vi "CRYCalculation TS Tree RowNum.vi"(0 "Tree Task SequenceIn":refnum<vi>, 5 "sOption":string) -> (3 "DispInfo Cluster Out":T1, 4 "Tree Task Sequence Out":refnum<vi>, 6 "SourceRowNum":i32, 8 "SourceCount":i32, 10 "TargetRowNum":i32, 14 "MoveCount":i32, 15 "EditRowNum":i32)   [LabVIEW 2013]
uses:
  CRYProject Editor Global.vi
panel:
  # "Insert new step into Project window."
  # "for Tree"
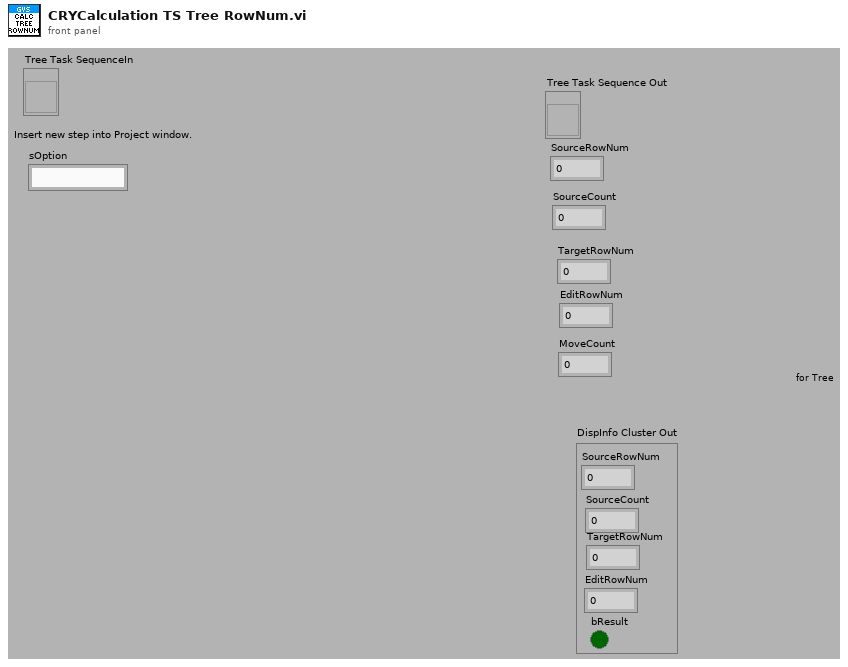
[diagram p1: front panel]
types:
  T1 = cluster{"SourceRowNum":i32, "SourceCount":i32, "TargetRowNum":i32, "bResult":bool, "EditRowNum":i32}
  T2 = typedef "CRYTS.ctl" = cluster{"No.TS":u16, "TS File Path":path, "TS Name":string, "EditStepName":string, "Steps":T3[], "New State":bool, "Change State":bool, "Flattened CurveLib Data":string, "Document Data":string, "EditStepNo":u16, "Operator Start File":string, "Sequence Type":string, "Sequence Language":string}
  T3 = typedef "CRYStep.ctl" = cluster{"No.VI":i32, "Category":string, "StepName":string, "Seq setup flattened":string, "Comment":string, "Steps config.":bool[], "Jump config":i32[], "Start":dbl, "Increment":dbl, "Name":string, "Unit":string, "Y data":u16, "Y prefix":string, "Y dB ref":dbl, "Y unit":string, "Repeat State Array":cluster{"Start":dbl, "Increment":dbl, "Count":i32, "Num":i32}[]}
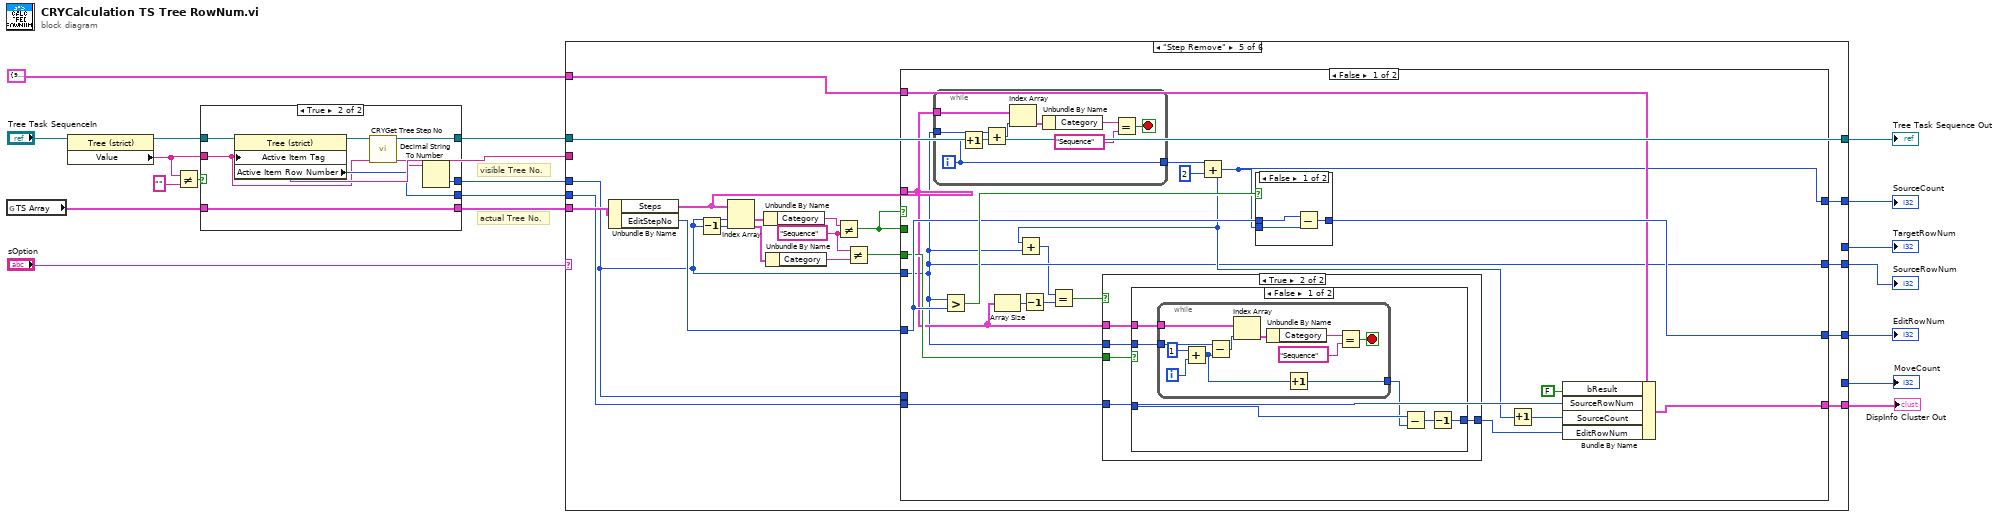
[diagram p0: block diagram]
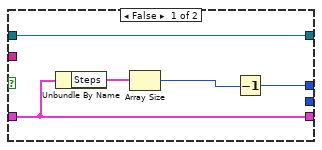
[diagram p2: hidden frame]
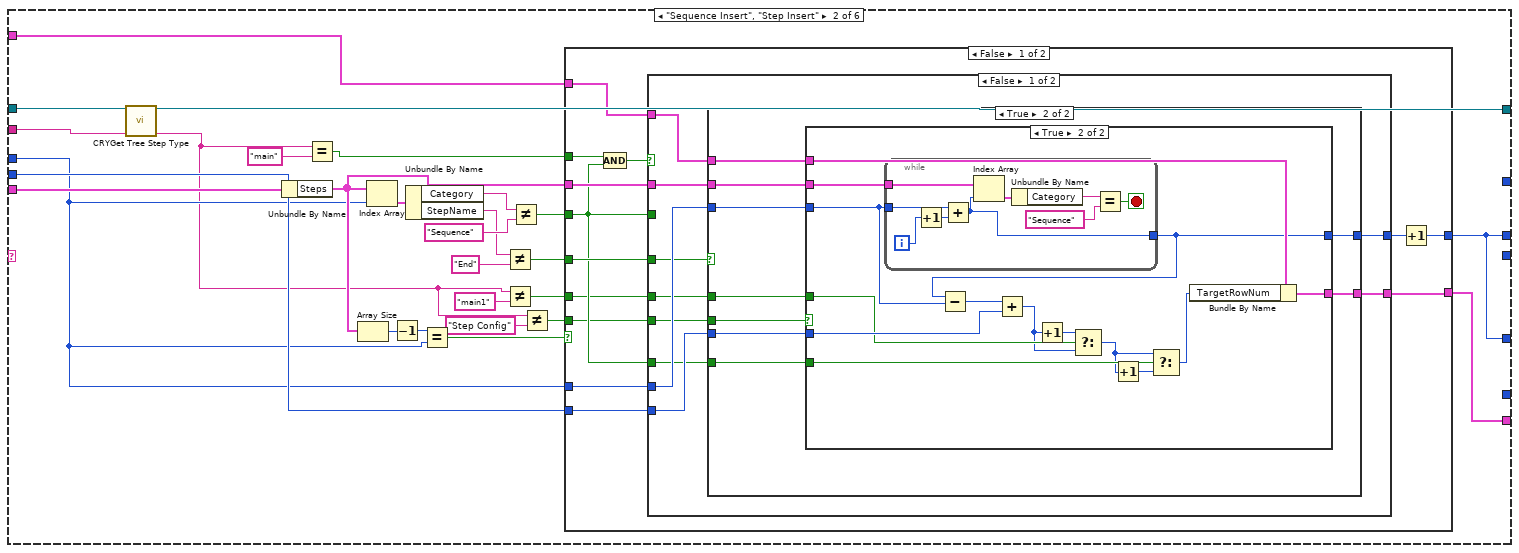
[diagram p4: hidden frame]
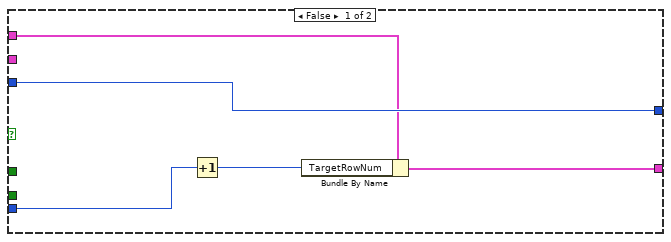
[diagram p5: hidden frame]
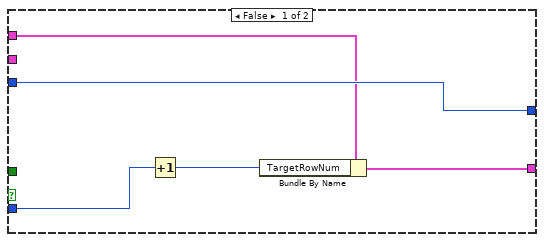
[diagram p6: hidden frame]
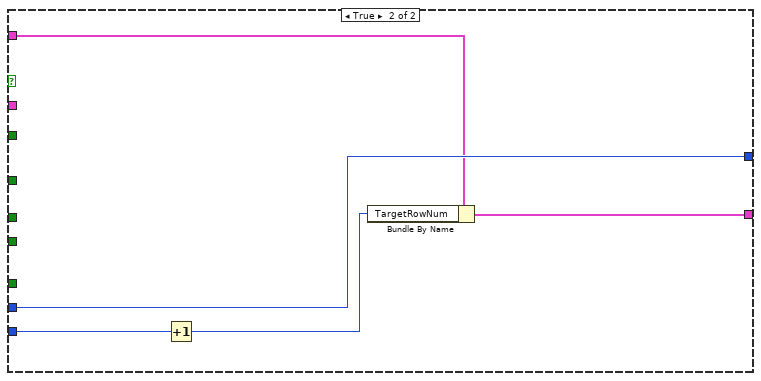
[diagram p7: hidden frame]
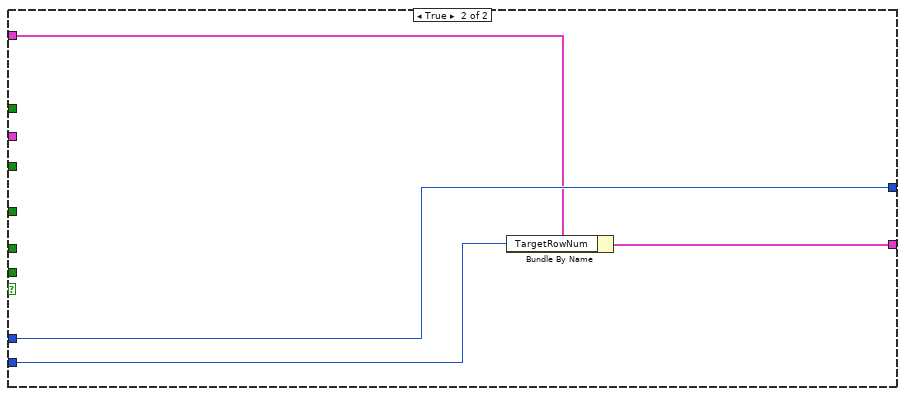
[diagram p8: hidden frame]
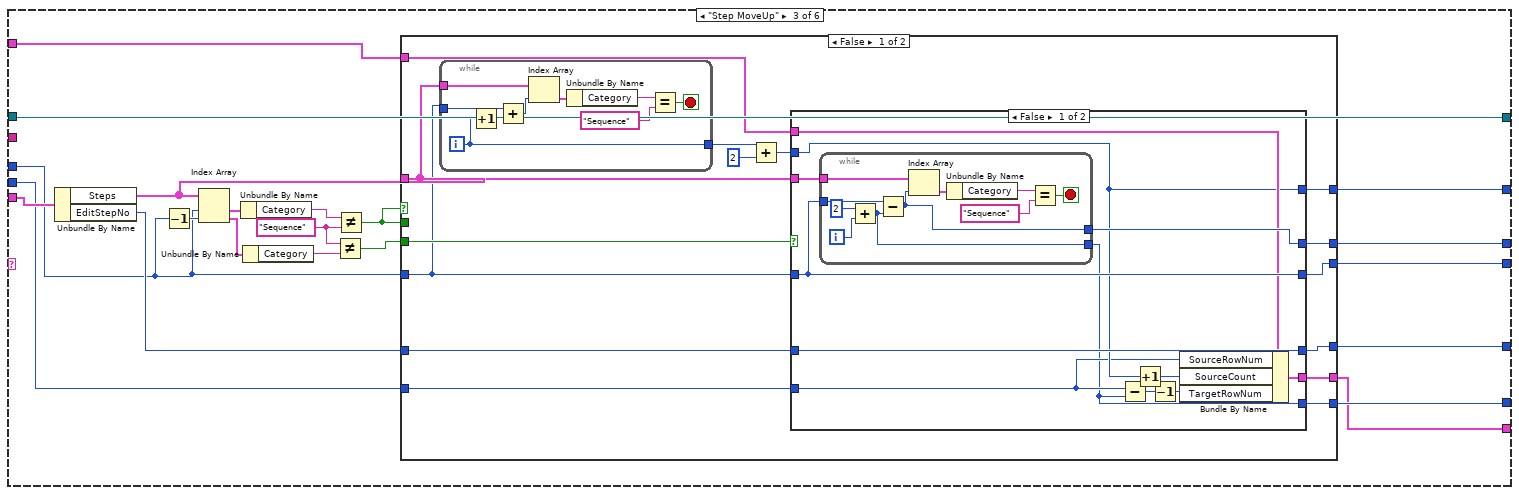
[diagram p9: hidden frame]
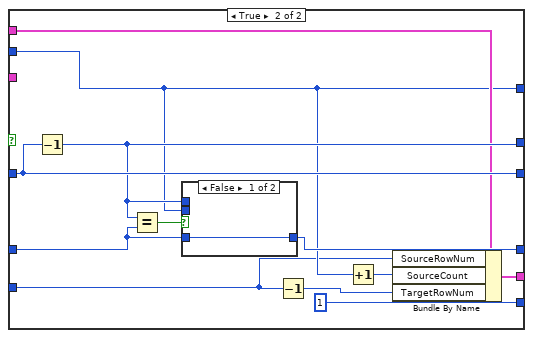
[diagram p10: hidden frame]
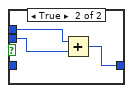
[diagram p11: hidden frame]
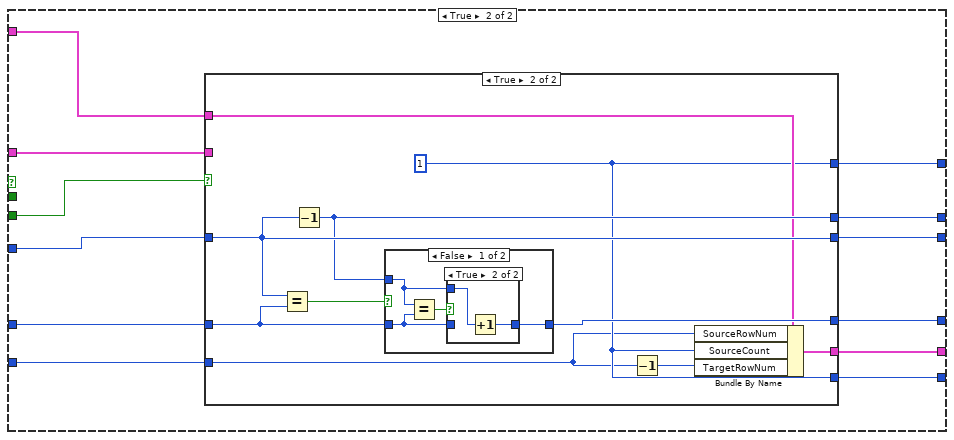
[diagram p12: hidden frame]
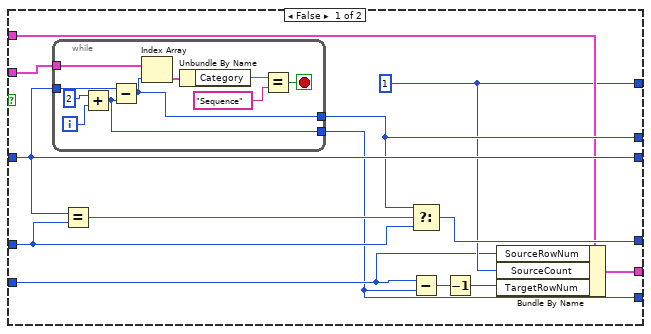
[diagram p13: hidden frame]
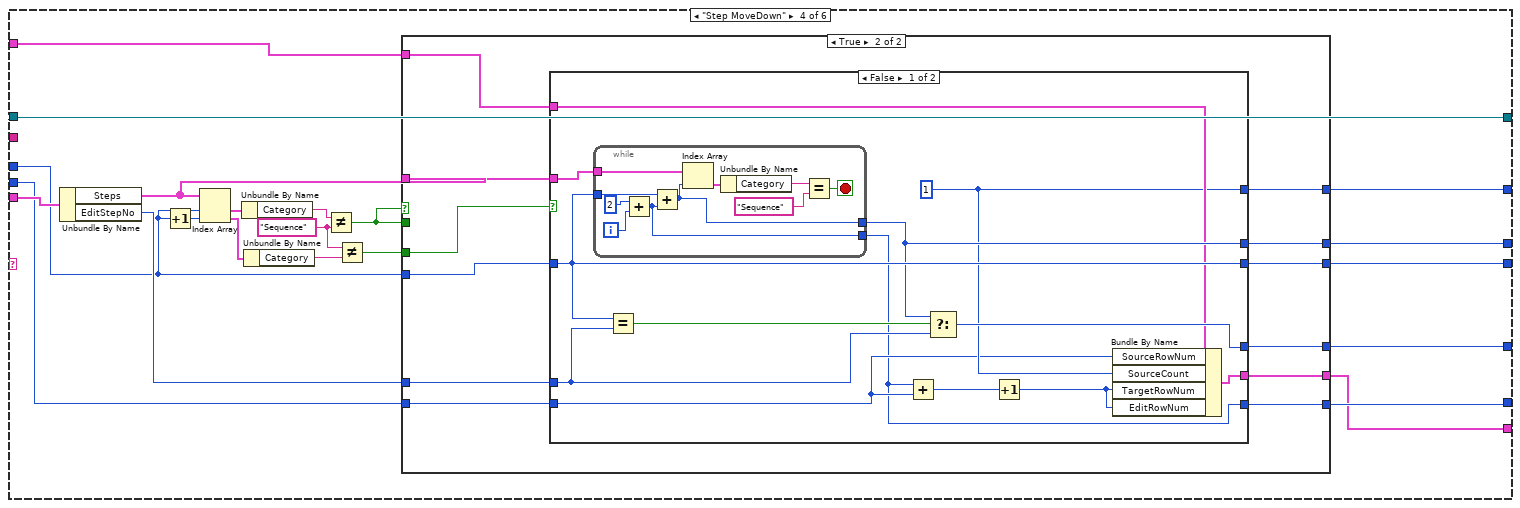
[diagram p16: hidden frame]
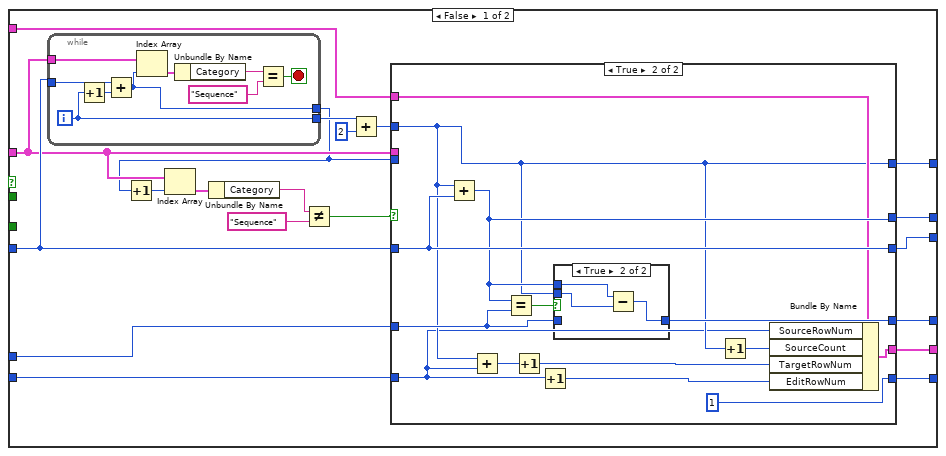
[diagram p17: hidden frame]
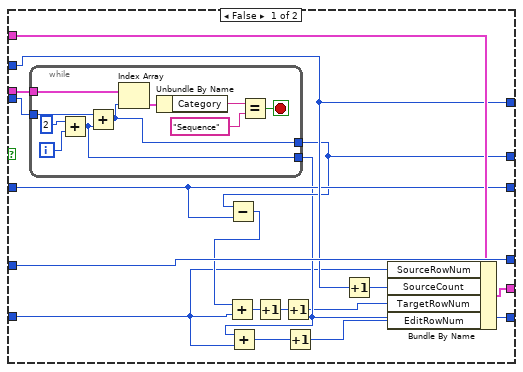
[diagram p18: hidden frame]
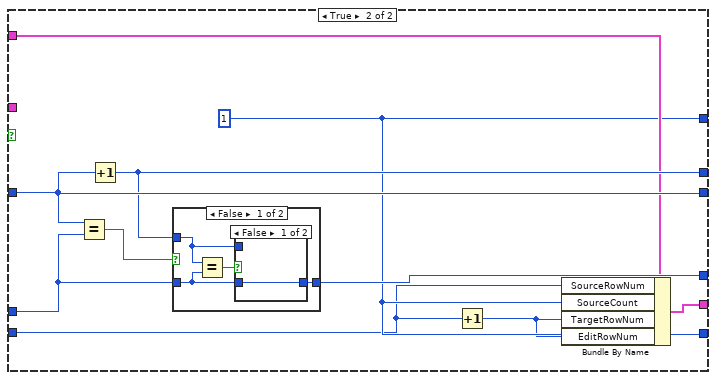
[diagram p20: hidden frame]
diagram:
  # "actual Tree No."
  # "visible Tree No."
  n1 = global read "CRYProject Editor Global.vi" "TS Array"() -> (w2:T2)
  n2 = property class="Tree (strict)"(reference="Tree Task SequenceIn") -> (reference out=w7:refnum<vi>, "Value"=w5:string)  [unwired: 1 in, 1 out]
  n3 = Not Equal?(x=w5, y="") -> (x != y?=w3:bool)
  n4 = case shown="True" w3 {
    tunnel: [w22 w32] -> w9
    tunnel: [_ w31] -> w8
    tunnel: w7 -> [w20 w29]
    tunnel: [w20 w27] -> w6
    tunnel: w5 -> [_ w26]
    tunnel: w2 -> [w21 w25]
    tunnel: [w21 w25] -> w1
    frame False {
      n5 = Unbundle By Name(w21) -> ("Steps"=w24:T3[])
      n6 = Array Size(array=w24) -> (size(s)=w23:i32)
      n7 = Decrement(x=w23) -> (x-1=w22:i32)
    }
    frame True {
      n8 = property class="Tree (strict)"(reference=w29, "Active Item Tag"=w26) -> (reference out=w28:refnum<vi>, "Active Item Row Number"=w31:i32)  [unwired: 1 in, 1 out]
      n9 = call "CRYGet Tree Step No.vi"("SequenceTree"=w28, "Active Item Tag"=w26) -> ("reference out"=w27:refnum<vi>, "Active Cell String4"=w30:string)  [unwired: 12 in]
      n10 = Decimal String To Number(string=w30) -> (number=w32:i32)  [unwired: 2 in, 1 out]
    }
  }
  n11 = case shown="\"Step Remove\"" "sOption" {
    tunnel: w6 -> [w33 w37 w135 w271 w420 w699]
    tunnel: [w33 w36 w135 w271 w420 w699] -> w19
    tunnel: [_ w49 w152 w288 _ _] -> w17
    tunnel: [_ _ w145 w281 w428 _] -> w16
    tunnel: [_ _ w144 w280 w427 _] -> w15
    tunnel: [_ w49 w143 w278 w425 _] -> w14
    tunnel: [_ _ w141 w277 _ _] -> w13
    tunnel: [_ w47 w139 w275 w424 w697] -> w12
    tunnel: T1 {"SourceRowNum"=9, "SourceCount"=19, "TargetRowNum"=42, "bResult"=FALSE, "EditRowNum"=42} ("DispInfo Cluster Out") -> [_ w48 w140 w276 w423 w698]
    tunnel: w1 -> [_ w42 w138 w274 w422 _]
    tunnel: w9 -> [_ w40 w136 w272 w419 w696]
    tunnel: w8 -> [_ w41 w137 w273 w421 _]
    tunnel: w5 -> [_ w35 _ _ _ _]
    frame Default {
    }
    frame "Sequence Insert", "Step Insert" {
      n12 = call "CRYGet Tree Step Type.vi"("SequenceTree"=w37, "Active Item Tag"=w35) -> ("reference out"=w36:refnum<vi>, "Active Cell String3"=w34:string)  [unwired: 12 in]
      n13 = Unbundle By Name(w42) -> ("Steps"=w55:T3[])
      n14 = Equal?(x=w34, y="main" ("decimal integer string")) -> (x = y?=w57:bool)
      n15 = Array Size(array=w55) -> (size(s)=w54:i32)
      n16 = Index Array(array=w55, index=w40) -> (element=w60:T3)
      n17 = Decrement(x=w54) -> (x-1=w53:i32)
      n18 = Unbundle By Name(w60) -> ("Category"=w59:string, "StepName"=w46:string)
      n19 = Equal?(x=w53, y=w40) -> (x = y?=w52:bool)
      n20 = Not Equal?(x=w46, y="End") -> (x != y?=w50:bool)
      n21 = Not Equal?(x=w34, y="main1" ("decimal integer string")) -> (x != y?=w45:bool)
      n22 = Not Equal?(x=w59, y="Sequence") -> (x != y?=w56:bool)
      n23 = Not Equal?(x=w34, y="Step Config" ("SequenceName")) -> (x != y?=w38:bool)
      n24 = case shown="False" w52 {
        tunnel: w57 -> [w73 _]
        tunnel: w56 -> [w63 _]
        tunnel: [w70 w134] -> w49
        tunnel: w55 -> [w69 _]
        tunnel: w40 -> [w68 w134]
        tunnel: w50 -> [w67 _]
        tunnel: w48 -> [w66 w133]
        tunnel: w41 -> [w65 w132]
        tunnel: [w64 w131] -> w47
        tunnel: w45 -> [w62 _]
        tunnel: w38 -> [w61 _]
        frame False {
          n25 = Compound Arithmetic op=AND(w73, w63) -> (w72:bool)
          n26 = case shown="False" w72 {
            tunnel: w68 -> [w83 w130]
            tunnel: w63 -> [_ _]
            tunnel: w69 -> [w82 _]
            tunnel: [w81 w130] -> w71
            tunnel: w67 -> [w80 _]
            tunnel: w66 -> [w79 w129]
            tunnel: w65 -> [w78 w128]
            tunnel: [w77 w127] -> w64
            tunnel: w63 -> [w76 _]
            tunnel: w62 -> [w75 _]
            tunnel: w61 -> [w74 _]
            frame False {
              n27 = case shown="True" w80 {
                tunnel: w83 -> [w88 w93]
                tunnel: w82 -> [_ w97]
                tunnel: [w88 w94] -> w81
                tunnel: w79 -> [w87 w96]
                tunnel: w78 -> [w86 w92]
                tunnel: [w85 w95] -> w77
                tunnel: w76 -> [_ w91]
                tunnel: w75 -> [_ w90]
                tunnel: w74 -> [_ w89]
                frame False {
                  n28 = Increment(x=w86) -> (x+1=w84:i32)
                  n29 = Bundle By Name(cluster=w87, "TargetRowNum"=w84) -> (w85:T1)
                }
                frame True {
                  n30 = case shown="True" w89 {
                    tunnel: w97 -> [_ w116]
                    tunnel: w96 -> [w100 w115]
                    tunnel: [w98 w114] -> w95
                    tunnel: [w101 w113] -> w94
                    tunnel: w93 -> [w101 w112]
                    tunnel: w92 -> [w99 w110]
                    tunnel: w91 -> [_ w109]
                    tunnel: w90 -> [_ w106]
                    frame False {
                      n31 = Increment(x=w99) -> (x+1=w102:i32)
                      n32 = Bundle By Name(cluster=w100, "TargetRowNum"=w102) -> (w98:T1)
                    }
                    frame True {
                      n33 = while {
                        tunnel: w116 -> [w125]
                        tunnel: w112 -> [w124]
                        tunnel: [w117] -> w113
                        i -> [w123]
                        stop <- w118 stop-if-true
                        n34 = Increment(x=w123) -> (x+1=w122:i32)
                        n35 = Add(x=w124, y=w122) -> (x+y=w117:i32)
                        n36 = Index Array(array=w125, index=w117) -> (element=w121:T3)
                        n37 = Unbundle By Name(w121) -> ("Category"=w120:string)
                        n38 = Equal?(x=w120, y="Sequence") -> (x = y?=w118:bool)
                      }
                      n39 = Subtract(x=w113, y=w112) -> (x-y=w111:i32)
                      n40 = Add(x=w111, y=w110) -> (x+y=w105:i32)
                      n41 = Increment(x=w105) -> (x+1=w104:i32)
                      n42 = Select(t=w104, s=w106, f=w105) -> (s? t:f=w103:i32)
                      n43 = Increment(x=w103) -> (x+1=w108:i32)
                      n44 = Select(t=w103, s=w109, f=w108) -> (s? t:f=w107:i32)
                      n45 = Bundle By Name(cluster=w115, "TargetRowNum"=w107) -> (w114:T1)
                    }
                  }
                }
              }
            }
            frame True {
              n46 = Increment(x=w128) -> (x+1=w126:i32)
              n47 = Bundle By Name(cluster=w129, "TargetRowNum"=w126) -> (w127:T1)
            }
          }
          n48 = Increment(x=w71) -> (x+1=w70:i32)
        }
        frame True {
          n49 = Bundle By Name(cluster=w133, "TargetRowNum"=w132) -> (w131:T1)
        }
      }
    }
    frame "Step MoveUp" {
      w147 = "Sequence" ("y")
      n50 = Unbundle By Name(w138) -> ("Steps"=w153:T3[], "EditStepNo"=w142:u16)
      n51 = Decrement(x=w136) -> (x-1=w150:i32)
      n52 = Index Array(array=w153, index #1=w136, index #2=w150) -> (element #1=w155:T3, element #2=w149:T3)
      n53 = Unbundle By Name(w155) -> ("Category"=w154:string)
      n54 = Unbundle By Name(w149) -> ("Category"=w148:string)
      n55 = Not Equal?(x=w147, y=w148) -> (x != y?=w146:bool)
      n56 = Not Equal?(x=w154, y=w147) -> (x != y?=w151:bool)
      n57 = case shown="False" w151 {
        tunnel: w136 -> [w165 w228]
        tunnel: w151 -> [_ _]
        tunnel: w153 -> [w166 w226]
        tunnel: [w170 w227] -> w152
        tunnel: w146 -> [w169 w229]
        tunnel: [w168 w225] -> w145
        tunnel: [w167 w224] -> w144
        tunnel: [w160 w223] -> w143
        tunnel: w142 -> [w161 w222]
        tunnel: [w159 w221] -> w141
        tunnel: w140 -> [w158 w220]
        tunnel: w137 -> [w157 w218]
        tunnel: [w156 w219] -> w139
        frame False {
          n58 = while {
            tunnel: w166 -> [w179]
            tunnel: w165 -> [w178]
            tunnel: [w171] -> w163
            i -> [w171]
            stop <- w173 stop-if-true
            n59 = Increment(x=w171) -> (x+1=w177:i32)
            n60 = Add(x=w178, y=w177) -> (x+y=w172:i32)
            n61 = Index Array(array=w179, index=w172) -> (element=w176:T3)
            n62 = Unbundle By Name(w176) -> ("Category"=w175:string)
            n63 = Equal?(x=w175, y="Sequence") -> (x = y?=w173:bool)
          }
          n64 = Add(x=w163, y=2) -> (x+y=w162:i32)
          n65 = case shown="False" w169 {
            tunnel: w166 -> [w191 _]
            tunnel: [w190 w211] -> w170
            tunnel: w165 -> [w189 w213]
            tunnel: [w189 w213] -> w168
            tunnel: [w186 w205] -> w167
            tunnel: w162 -> [w186 w205]
            tunnel: w161 -> [w188 w210]
            tunnel: [w188 w209] -> w160
            tunnel: [w183 1] -> w159
            tunnel: w158 -> [w187 w207]
            tunnel: w157 -> [w184 w203]
            tunnel: [w180 w206] -> w156
            frame False {
              n66 = while {
                tunnel: w191 -> [w201]
                tunnel: w189 -> [w200]
                tunnel: [w195] -> w190
                tunnel: [w192] -> w183
                i -> [w194]
                stop <- w196 stop-if-true
                n67 = Add(x=2, y=w194) -> (x+y=w192:i32)
                n68 = Subtract(x=w200, y=w192) -> (x-y=w195:i32)
                n69 = Index Array(array=w201, index=w195) -> (element=w199:T3)
                n70 = Unbundle By Name(w199) -> ("Category"=w198:string)
                n71 = Equal?(x=w198, y="Sequence") -> (x = y?=w196:bool)
              }
              n72 = Subtract(x=w184, y=w183) -> (x-y=w182:i32)
              n73 = Increment(x=w186) -> (x+1=w185:i32)
              n74 = Decrement(x=w182) -> (x-1=w181:i32)
              n75 = Bundle By Name(cluster=w187, "SourceRowNum"=w184, "SourceCount"=w185, "TargetRowNum"=w181) -> (w180:T1)
            }
            frame True {
              n76 = Decrement(x=w213) -> (x-1=w211:i32)
              n77 = Equal?(x=w211, y=w210) -> (x = y?=w212:bool)
              n78 = case shown="False" w212 {
                tunnel: w211 -> [_ w217]
                tunnel: [w214 w215] -> w209
                tunnel: w210 -> [w214 _]
                tunnel: w205 -> [_ w216]
                frame False {
                }
                frame True {
                  n79 = Add(x=w217, y=w216) -> (x+y=w215:i32)
                }
              }
              n80 = Decrement(x=w203) -> (x-1=w202:i32)
              n81 = Increment(x=w205) -> (x+1=w204:i32)
              n82 = Bundle By Name(cluster=w207, "SourceRowNum"=w203, "SourceCount"=w204, "TargetRowNum"=w202) -> (w206:T1)
            }
          }
        }
        frame True {
          n83 = case shown="True" w229 {
            tunnel: [w239 w260] -> w227
            tunnel: w228 -> [w241 w262]
            tunnel: w226 -> [w242 _]
            tunnel: [w241 w262] -> w225
            tunnel: [w234 w255] -> w224
            tunnel: [w237 w259] -> w223
            tunnel: w222 -> [w238 w258]
            tunnel: [w232 w255] -> w221
            tunnel: w220 -> [w236 w257]
            tunnel: [w235 w256] -> w219
            tunnel: w218 -> [w233 w254]
            frame False {
              w234 = 1 ("x-1")
              n84 = while {
                tunnel: w242 -> [w252]
                tunnel: w241 -> [w251]
                tunnel: [w246] -> w239
                tunnel: [w243] -> w232
                i -> [w245]
                stop <- w247 stop-if-true
                n85 = Add(x=2, y=w245) -> (x+y=w243:i32)
                n86 = Subtract(x=w251, y=w243) -> (x-y=w246:i32)
                n87 = Index Array(array=w252, index=w246) -> (element=w250:T3)
                n88 = Unbundle By Name(w250) -> ("Category"=w249:string)
                n89 = Equal?(x=w249, y="Sequence") -> (x = y?=w247:bool)
              }
              n90 = Equal?(x=w241, y=w238) -> (x = y?=w240:bool)
              n91 = Select(t=w239, s=w240, f=w238) -> (s? t:f=w237:i32)
              n92 = Subtract(x=w233, y=w232) -> (x-y=w231:i32)
              n93 = Decrement(x=w231) -> (x-1=w230:i32)
              n94 = Bundle By Name(cluster=w236, "SourceRowNum"=w233, "SourceCount"=w234, "TargetRowNum"=w230) -> (w235:T1)
            }
            frame True {
              w255 = 1 ("x-1")
              n95 = Equal?(x=w262, y=w258) -> (x = y?=w261:bool)
              n96 = Decrement(x=w262) -> (x-1=w260:i32)
              n97 = case shown="False" w261 {
                tunnel: [w264 w270] -> w259
                tunnel: w260 -> [w265 w270]
                tunnel: w258 -> [w263 _]
                frame False {
                  n98 = Equal?(x=w265, y=w263) -> (x = y?=w266:bool)
                  n99 = case shown="True" w266 {
                    tunnel: w265 -> [_ w269]
                    tunnel: [w267 w268] -> w264
                    tunnel: w263 -> [w267 _]
                    frame False {
                    }
                    frame True {
                      n100 = Increment(x=w269) -> (x+1=w268:i32)
                    }
                  }
                }
                frame True {
                }
              }
              n101 = Decrement(x=w254) -> (x-1=w253:i32)
              n102 = Bundle By Name(cluster=w257, "SourceRowNum"=w254, "SourceCount"=w255, "TargetRowNum"=w253) -> (w256:T1)
            }
          }
        }
      }
    }
    frame "Step MoveDown" {
      w283 = "Sequence" ("y")
      n103 = Unbundle By Name(w274) -> ("Steps"=w289:T3[], "EditStepNo"=w279:u16)
      n104 = Increment(x=w272) -> (x+1=w286:i32)
      n105 = Index Array(array=w289, index #1=w272, index #2=w286) -> (element #1=w291:T3, element #2=w285:T3)
      n106 = Unbundle By Name(w291) -> ("Category"=w290:string)
      n107 = Unbundle By Name(w285) -> ("Category"=w284:string)
      n108 = Not Equal?(x=w290, y=w283) -> (x != y?=w287:bool)
      n109 = Not Equal?(x=w283, y=w284) -> (x != y?=w282:bool)
      n110 = case shown="True" w287 {
        tunnel: w272 -> [w308 w376]
        tunnel: w287 -> [_ _]
        tunnel: w289 -> [w301 w374]
        tunnel: [w311 w375] -> w288
        tunnel: w282 -> [_ w377]
        tunnel: [w310 w373] -> w281
        tunnel: [w309 w372] -> w280
        tunnel: w279 -> [w305 w371]
        tunnel: [w304 w370] -> w278
        tunnel: [w303 w369] -> w277
        tunnel: w276 -> [w294 w368]
        tunnel: w273 -> [w293 w366]
        tunnel: [w292 w367] -> w275
        frame False {
          n111 = while {
            tunnel: w301 -> [w320]
            tunnel: w308 -> [w319]
            tunnel: [w313] -> w300
            tunnel: [w312] -> w295
            i -> [w313]
            stop <- w314 stop-if-true
            n112 = Increment(x=w313) -> (x+1=w318:i32)
            n113 = Add(x=w319, y=w318) -> (x+y=w312:i32)
            n114 = Index Array(array=w320, index=w312) -> (element=w317:T3)
            n115 = Unbundle By Name(w317) -> ("Category"=w316:string)
            n116 = Equal?(x=w316, y="Sequence") -> (x = y?=w314:bool)
          }
          n117 = Increment(x=w295) -> (x+1=w299:i32)
          n118 = Index Array(array=w301, index=w299) -> (element=w302:T3)
          n119 = Unbundle By Name(w302) -> ("Category"=w298:string)
          n120 = Not Equal?(x=w298, y="Sequence") -> (x != y?=w296:bool)
          n121 = Add(x=w300, y=2) -> (x+y=w306:i32)
          n122 = case shown="True" w296 {
            tunnel: w301 -> [w337 _]
            tunnel: [w327 w356] -> w311
            tunnel: w308 -> [w329 w358]
            tunnel: [w329 w358] -> w310
            tunnel: [w332 w352] -> w309
            tunnel: w306 -> [w332 w352]
            tunnel: [w336 w360] -> w304
            tunnel: w305 -> [w336 w361]
            tunnel: [w326 1] -> w303
            tunnel: w295 -> [w335 _]
            tunnel: w294 -> [w334 w355]
            tunnel: w293 -> [w325 w349]
            tunnel: [w333 w353] -> w292
            frame False {
              n123 = while {
                tunnel: w337 -> [w347]
                tunnel: w335 -> [w346]
                tunnel: [w341] -> w327
                tunnel: [w338] -> w326
                i -> [w340]
                stop <- w342 stop-if-true
                n124 = Add(x=2, y=w340) -> (x+y=w338:i32)
                n125 = Add(x=w346, y=w338) -> (x+y=w341:i32)
                n126 = Index Array(array=w347, index=w341) -> (element=w345:T3)
                n127 = Unbundle By Name(w345) -> ("Category"=w344:string)
                n128 = Equal?(x=w344, y="Sequence") -> (x = y?=w342:bool)
              }
              n129 = Subtract(x=w327, y=w329) -> (x-y=w328:i32)
              n130 = Add(x=w328, y=w325) -> (x+y=w330:i32)
              n131 = Add(x=w326, y=w325) -> (x+y=w322:i32)
              n132 = Increment(x=w330) -> (x+1=w324:i32)
              n133 = Increment(x=w324) -> (x+1=w323:i32)
              n134 = Increment(x=w322) -> (x+1=w321:i32)
              n135 = Increment(x=w332) -> (x+1=w331:i32)
              n136 = Bundle By Name(cluster=w334, "SourceRowNum"=w325, "SourceCount"=w331, "TargetRowNum"=w323, "EditRowNum"=w321) -> (w333:T1)
            }
            frame True {
              n137 = Add(x=w352, y=w358) -> (x+y=w356:i32)
              n138 = Add(x=w352, y=w349) -> (x+y=w351:i32)
              n139 = Equal?(x=w356, y=w361) -> (x = y?=w359:bool)
              n140 = Increment(x=w351) -> (x+1=w350:i32)
              n141 = Increment(x=w349) -> (x+1=w348:i32)
              n142 = case shown="True" w359 {
                tunnel: w356 -> [_ w365]
                tunnel: [w362 w363] -> w360
                tunnel: w361 -> [w362 _]
                tunnel: w352 -> [_ w364]
                frame False {
                }
                frame True {
                  n143 = Subtract(x=w365, y=w364) -> (x-y=w363:i32)
                }
              }
              n144 = Increment(x=w352) -> (x+1=w354:i32)
              n145 = Bundle By Name(cluster=w355, "SourceRowNum"=w349, "SourceCount"=w354, "TargetRowNum"=w350, "EditRowNum"=w348) -> (w353:T1)
            }
          }
        }
        frame True {
          n146 = case shown="False" w377 {
            tunnel: [w385 w406] -> w375
            tunnel: w376 -> [w389 w410]
            tunnel: w374 -> [w390 _]
            tunnel: [w389 w410] -> w373
            tunnel: [w382 w403] -> w372
            tunnel: w371 -> [w387 w408]
            tunnel: [w386 w407] -> w370
            tunnel: [w380 w403] -> w369
            tunnel: w368 -> [w384 w405]
            tunnel: [w383 w404] -> w367
            tunnel: w366 -> [w381 w402]
            frame False {
              w382 = 1 ("x-1")
              n147 = while {
                tunnel: w390 -> [w400]
                tunnel: w389 -> [w399]
                tunnel: [w394] -> w385
                tunnel: [w391] -> w380
                i -> [w393]
                stop <- w395 stop-if-true
                n148 = Add(x=2, y=w393) -> (x+y=w391:i32)
                n149 = Add(x=w399, y=w391) -> (x+y=w394:i32)
                n150 = Index Array(array=w400, index=w394) -> (element=w398:T3)
                n151 = Unbundle By Name(w398) -> ("Category"=w397:string)
                n152 = Equal?(x=w397, y="Sequence") -> (x = y?=w395:bool)
              }
              n153 = Equal?(x=w389, y=w387) -> (x = y?=w388:bool)
              n154 = Add(x=w380, y=w381) -> (x+y=w379:i32)
              n155 = Select(t=w385, s=w388, f=w387) -> (s? t:f=w386:i32)
              n156 = Increment(x=w379) -> (x+1=w378:i32)
              n157 = Bundle By Name(cluster=w384, "SourceRowNum"=w381, "SourceCount"=w382, "TargetRowNum"=w378, "EditRowNum"=w378) -> (w383:T1)
            }
            frame True {
              w403 = 1 ("x-1")
              n158 = Equal?(x=w410, y=w408) -> (x = y?=w409:bool)
              n159 = Increment(x=w410) -> (x+1=w406:i32)
              n160 = case shown="False" w409 {
                tunnel: [w412 w418] -> w407
                tunnel: w406 -> [w413 w418]
                tunnel: w408 -> [w411 _]
                frame False {
                  n161 = Equal?(x=w413, y=w411) -> (x = y?=w414:bool)
                  n162 = case shown="False" w414 {
                    tunnel: w413 -> [_ w417]
                    tunnel: [w415 w416] -> w412
                    tunnel: w411 -> [w415 _]
                    frame False {
                    }
                    frame True {
                      n163 = Decrement(x=w417) -> (x-1=w416:i32)
                    }
                  }
                }
                frame True {
                }
              }
              n164 = Increment(x=w402) -> (x+1=w401:i32)
              n165 = Bundle By Name(cluster=w405, "SourceRowNum"=w402, "SourceCount"=w403, "TargetRowNum"=w401, "EditRowNum"=w401) -> (w404:T1)
            }
          }
        }
      }
    }
    frame "Step Remove" {
      w430 = "Sequence" ("y")
      n166 = Unbundle By Name(w422) -> ("Steps"=w435:T3[], "EditStepNo"=w426:u16)
      n167 = Decrement(x=w419) -> (x-1=w433:i32)
      n168 = Index Array(array=w435, index #1=w419, index #2=w433) -> (element #1=w437:T3, element #2=w432:T3)
      n169 = Unbundle By Name(w437) -> ("Category"=w436:string)
      n170 = Unbundle By Name(w432) -> ("Category"=w431:string)
      n171 = Not Equal?(x=w436, y=w430) -> (x != y?=w434:bool)
      n172 = Not Equal?(x=w430, y=w431) -> (x != y?=w429:bool)
      n173 = case shown="False" w434 {
        tunnel: w419 -> [w441 w500]
        tunnel: w434 -> [_ _]
        tunnel: w435 -> [w444 w499]
        tunnel: w429 -> [w446 w498]
        tunnel: [w441 w500] -> w428
        tunnel: [w442 w501] -> w427
        tunnel: w426 -> [w453 w506]
        tunnel: [w452 w508] -> w425
        tunnel: [w449 w504] -> w424
        tunnel: w423 -> [w451 w503]
        tunnel: w421 -> [w447 w497]
        tunnel: w419 -> [_ w495]
        frame False {
          n174 = while {
            tunnel: w444 -> [w494]
            tunnel: w441 -> [w493]
            tunnel: [w486] -> w455
            i -> [w486]
            stop <- w488 stop-if-true
            n175 = Increment(x=w486) -> (x+1=w492:i32)
            n176 = Add(x=w493, y=w492) -> (x+y=w487:i32)
            n177 = Index Array(array=w494, index=w487) -> (element=w491:T3)
            n178 = Unbundle By Name(w491) -> ("Category"=w490:string)
            n179 = Equal?(x=w490, y="Sequence") -> (x = y?=w488:bool)
          }
          n180 = Greater?(x=w441, y=w453) -> (0:w454:bool)
          n181 = Array Size(array=w444) -> (size(s)=w443:i32)
          n182 = Decrement(x=w443) -> (x-1=w440:i32)
          n183 = Add(x=w455, y=2) -> (x+y=w442:i32)
          n184 = Add(x=w442, y=w441) -> (x+y=w439:i32)
          n185 = Equal?(x=w439, y=w440) -> (x = y?=w438:bool)
          n186 = case shown="True" w438 {
            tunnel: w447 -> [w457 w462]
            tunnel: w446 -> [_ w461]
            tunnel: [w457 w460] -> w445
            tunnel: w444 -> [_ w459]
            tunnel: w441 -> [_ w458]
            frame False {
            }
            frame True {
              n187 = case shown="False" w461 {
                tunnel: w459 -> [w468 _]
                tunnel: w458 -> [w467 _]
                tunnel: w462 -> [w466 w481]
                tunnel: [w463 w480] -> w460
                frame False {
                  n188 = while {
                    tunnel: w468 -> [w479]
                    tunnel: w467 -> [w478]
                    tunnel: [w469] -> w465
                    i -> [w472]
                    stop <- w474 stop-if-true
                    n189 = Add(x=1, y=w472) -> (x+y=w470:i32)
                    n190 = Subtract(x=w478, y=w470) -> (x-y=w473:i32)
                    n191 = Index Array(array=w479, index=w473) -> (element=w477:T3)
                    n192 = Unbundle By Name(w477) -> ("Category"=w476:string)
                    n193 = Increment(x=w470) -> (x+1=w469:i32)
                    n194 = Equal?(x=w476, y="Sequence") -> (x = y?=w474:bool)
                  }
                  n195 = Subtract(x=w466, y=w465) -> (x-y=w464:i32)
                  n196 = Decrement(x=w464) -> (x-1=w463:i32)
                }
                frame True {
                  n197 = Decrement(x=w481) -> (x-1=w480:i32)
                }
              }
            }
          }
          n198 = case shown="False" w454 {
            tunnel: [w483 w485] -> w452
            tunnel: w453 -> [w484 w485]
            tunnel: w442 -> [w482 _]
            frame False {
              n199 = Subtract(x=w484, y=w482) -> (x-y=w483:i32)
            }
            frame True {
            }
          }
          n200 = Increment(x=w442) -> (x+1=w448:i32)
          n201 = Bundle By Name(cluster=w451, "bResult"=FALSE, "SourceRowNum"=w447, "SourceCount"=w448, "EditRowNum"=w445) -> (w449:T1)
        }
        frame True {
          w501 = 1 ("x-1")
          n202 = Greater?(x=w500, y=w506) -> (0:w505:bool)
          n203 = Equal?(x=w500, y=w506) -> (x = y?=w507:bool)
          n204 = case shown="True" w507 {
            tunnel: [w519 w552] -> w508
            tunnel: w506 -> [w520 _]
            tunnel: w505 -> [w521 _]
            tunnel: [FALSE ("bResult") TRUE ("bResult")] -> w502
            tunnel: w500 -> [w511 w554]
            tunnel: w499 -> [w515 w555]
            tunnel: w498 -> [w517 _]
            tunnel: [w516 w551] -> w496
            tunnel: w495 -> [w509 w549]
            frame False {
              n205 = Array Size(array=w515) -> (size(s)=w514:i32)
              n206 = Subtract(x=w514, y=2) -> (x-y=w512:i32)
              n207 = Equal?(x=w512, y=w511) -> (x = y?=w510:bool)
              n208 = case shown="True" w521 {
                tunnel: [w546 w548] -> w519
                tunnel: w520 -> [w547 w548]
                frame False {
                  n209 = Decrement(x=w547) -> (x-1=w546:u16)
                }
                frame True {
                }
              }
              n210 = case shown="True" w510 {
                tunnel: w517 -> [_ w527]
                tunnel: w509 -> [w522 w526]
                tunnel: [w522 w525] -> w516
                tunnel: w515 -> [_ w524]
                tunnel: w511 -> [_ w523]
                frame False {
                }
                frame True {
                  n211 = case shown="True" w527 {
                    tunnel: w524 -> [w533 _]
                    tunnel: w523 -> [w532 _]
                    tunnel: w526 -> [w531 w545]
                    tunnel: [w528 w544] -> w525
                    frame False {
                      n212 = while {
                        tunnel: w533 -> [w543]
                        tunnel: w532 -> [w542]
                        tunnel: [w537] -> _
                        tunnel: [w534] -> w530
                        i -> [w536]
                        stop <- w538 stop-if-true
                        n213 = Add(x=2, y=w536) -> (x+y=w534:i32)
                        n214 = Subtract(x=w542, y=w534) -> (x-y=w537:i32)
                        n215 = Index Array(array=w543, index=w537) -> (element=w541:T3)
                        n216 = Unbundle By Name(w541) -> ("Category"=w540:string)
                        n217 = Equal?(x=w540, y="Sequence") -> (x = y?=w538:bool)
                      }
                      n218 = Subtract(x=w531, y=w530) -> (x-y=w529:i32)
                      n219 = Decrement(x=w529) -> (x-1=w528:i32)
                    }
                    frame True {
                      n220 = Decrement(x=w545) -> (x-1=w544:i32)
                    }
                  }
                }
              }
            }
            frame True {
              w553 = FALSE ("x != y?")
              n221 = while {
                tunnel: w555 -> [w568]
                shift-right: [w569] -> _
                shift-left: w553 -> [w570]
                tunnel: w554 -> [w566]
                shift-right: [w564] -> _
                shift-left: w553 -> [w565]
                shift-right: [w562] -> _
                shift-left: w553 -> [w563]
                shift-right: [w560] -> w551
                shift-left: w549 -> [w561]
                tunnel: [w559] -> w552
                shift-right: [w557] -> _
                shift-left: 0 ("Active Item Row Number") -> [w558]
                i -> [w571]
                stop <- w567 stop-if-true
                n222 = case shown="False" w565 {
                  selector: w565 -> [w582 w635]
                  tunnel: w571 -> [w593 w643]
                  tunnel: w570 -> [w591 w641]
                  tunnel: [w588 w639] -> w569
                  tunnel: w568 -> [w586 w637]
                  tunnel: [w580 w633] -> w567
                  tunnel: w566 -> [w583 w636]
                  tunnel: [w581 w634] -> w564
                  tunnel: w563 -> [w577 w628]
                  tunnel: [w578 w627] -> w562
                  tunnel: w561 -> [w576 w630]
                  tunnel: [w576 w629] -> w560
                  tunnel: [w572 w624] -> w559
                  tunnel: w558 -> [_ w622]
                  tunnel: [w573 w622] -> w557
                  frame False {
                    n223 = Increment(x=w593) -> (x+1=w573:i32)
                    n224 = Add(x=w583, y=w573) -> (x+y=w575:i32)
                    n225 = Index Array(array=w586, index=w575) -> (element=w595:T3)
                    n226 = Array Size(array=w586) -> (size(s)=w585:i32)
                    n227 = Unbundle By Name(w595) -> ("Category"=w574:string, "StepName"=w587:string)
                    n228 = Increment(x=w575) -> (x+1=w584:i32)
                    n229 = Equal?(x=w585, y=w584) -> (x = y?=w579:bool)
                    n230 = Equal?(x=w587, y="Start") -> (x = y?=w592:bool)
                    n231 = Equal?(x=w587, y="End") -> (x = y?=w589:bool)
                    n232 = case shown="False" w592 {
                      tunnel: w591 -> [w604 _]
                      tunnel: w589 -> [w605 _]
                      tunnel: [w603 TRUE ("x != y?")] -> w588
                      tunnel: w574 -> [w602 _]
                      tunnel: [w601 FALSE ("x != y?")] -> w580
                      tunnel: w582 -> [w600 w619]
                      tunnel: [w599 w619] -> w581
                      tunnel: w579 -> [w598 _]
                      tunnel: w577 -> [w597 _]
                      tunnel: [w596 TRUE ("x != y?")] -> w578
                      frame False {
                        n233 = case shown="True" w605 {
                          tunnel: w604 -> [w609 _]
                          tunnel: [w609 w617] -> w603
                          tunnel: w602 -> [w614 _]
                          tunnel: [w611 w617] -> w601
                          tunnel: w600 -> [w610 _]
                          tunnel: [w610 w616] -> w599
                          tunnel: w598 -> [_ w616]
                          tunnel: w597 -> [w607 w615]
                          tunnel: [w608 w615] -> w596
                          frame False {
                            n234 = Not Equal?(x=w614, y="Display") -> (x != y?=w612:bool)
                            n235 = Select(t=w607, s=w609, f=TRUE ("x != y?")) -> (s? t:f=w608:bool)
                            n236 = Compound Arithmetic op=AND(invert w609, w612) -> (w611:bool)
                          }
                          frame True {
                            w617 = FALSE ("x != y?")
                          }
                        }
                      }
                      frame True {
                      }
                    }
                    n237 = Decrement(x=w575) -> (x-1=w572:i32)
                  }
                  frame True {
                    n238 = Increment(x=w643) -> (x+1=w626:i32)
                    n239 = Subtract(x=w626, y=w622) -> (x-y=w623:i32)
                    n240 = Subtract(x=w636, y=w623) -> (x-y=w624:i32)
                    n241 = Index Array(array=w637, index=w624) -> (element=w644:T3)
                    n242 = Unbundle By Name(w644) -> ("Category"=w625:string, "StepName"=w638:string)
                    n243 = Equal?(x=w638, y="End") -> (x = y?=w642:bool)
                    n244 = Equal?(x=w638, y="Start") -> (x = y?=w640:bool)
                    n245 = case shown="False" w642 {
                      tunnel: w641 -> [w655 _]
                      tunnel: w640 -> [w656 _]
                      tunnel: [w654 TRUE ("x != y?")] -> w639
                      tunnel: w625 -> [w653 _]
                      tunnel: [w652 FALSE ("x != y?")] -> w633
                      tunnel: w635 -> [w651 w693]
                      tunnel: [w650 w693] -> w634
                      tunnel: w630 -> [w649 w692]
                      tunnel: [w645 w692] -> w629
                      tunnel: [w647 w691] -> w627
                      tunnel: w628 -> [w648 w691]
                      tunnel: w623 -> [w646 _]
                      frame False {
                        n246 = case shown="False" w656 {
                          tunnel: w655 -> [w657 _]
                          tunnel: [w657 w690] -> w654
                          tunnel: w653 -> [w668 _]
                          tunnel: [w665 w690] -> w652
                          tunnel: w651 -> [w664 w689]
                          tunnel: [w664 w689] -> w650
                          tunnel: w649 -> [w662 w686]
                          tunnel: w648 -> [w659 w685]
                          tunnel: [w658 TRUE ("x != y?")] -> w647
                          tunnel: w646 -> [w663 w687]
                          tunnel: [w660 w684] -> w645
                          frame False {
                            n247 = Subtract(x=w662, y=w663) -> (x-y=w661:i32)
                            n248 = Not Equal?(x=w668, y="Display") -> (x != y?=w666:bool)
                            n249 = case shown="False" w659 {
                              selector: w659 -> [w671 w679]
                              tunnel: w662 -> [w674 w680]
                              tunnel: w661 -> [w673 _]
                              tunnel: [w672 w680] -> w660
                              tunnel: [w669 w679] -> w658
                              tunnel: w657 -> [w670 _]
                              frame False {
                                n250 = case shown="False" w670 {
                                tunnel: w674 -> [_ w678]
                                tunnel: w673 -> [w676 _]
                                tunnel: [w676 w678] -> w672
                                tunnel: w671 -> [_ w677]
                                tunnel: [TRUE w677] -> w669
                                frame False {
                                }
                                frame True {
                                }
                                }
                              }
                              frame True {
                              }
                            }
                            n251 = Compound Arithmetic op=AND(invert w657, w666) -> (w665:bool)
                          }
                          frame True {
                            w690 = FALSE ("x != y?")
                            n252 = Subtract(x=w686, y=w687) -> (x-y=w688:i32)
                            n253 = Decrement(x=w688) -> (x-1=w681:i32)
                            n254 = Not(x=w685) -> (.not. x?=w682:bool)
                            n255 = Select(t=w681, s=w682, f=w686) -> (s? t:f=w684:i32)
                          }
                        }
                      }
                      frame True {
                      }
                    }
                  }
                }
              }
            }
          }
          n256 = Bundle By Name(cluster=w503, "bResult"=w502, "SourceRowNum"=w497, "SourceCount"=w501, "EditRowNum"=w496) -> (w504:T1)
        }
      }
    }
    frame "Step Configure" {
      n257 = Bundle By Name(cluster=w698, "EditRowNum"=w696) -> (w697:T1)
    }
  }
  "Tree Task Sequence Out" <- w19
  "TargetRowNum" <- w17
  "SourceRowNum" <- w16
  "SourceCount" <- w15
  "EditRowNum" <- w14
  "MoveCount" <- w13
  "DispInfo Cluster Out" <- w12
